vi "CRYGet Foot Switch.vi"(11 "Switch Mode":enum16{"ONESTOP_MODE", "CONTINUE_MODE"}(ring)) -> (3 "bResult":bool)   [LabVIEW 2013]
uses:
  CRYMainGlobal.vi
  Hardware/SubVI/CRY6175APT_Win32.dll
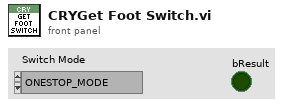
[diagram p1: front panel]
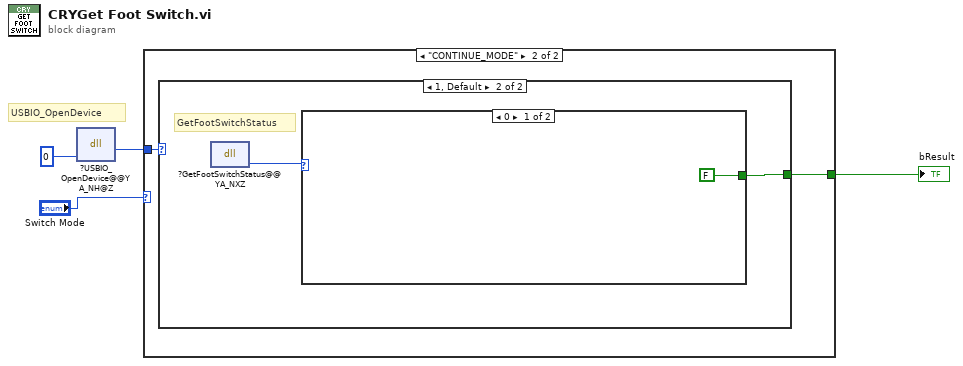
[diagram p0: block diagram]
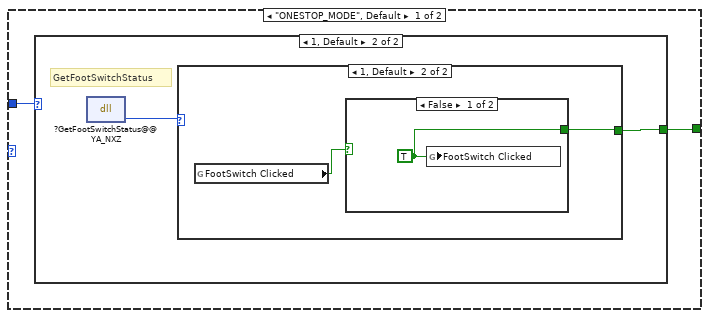
[diagram p2: hidden frame]
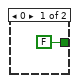
[diagram p3: hidden frame]
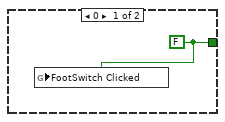
[diagram p4: hidden frame]
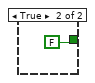
[diagram p5: hidden frame]
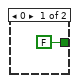
[diagram p6: hidden frame]
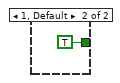
[diagram p7: hidden frame]
diagram:
  # "USBIO_OpenDevice"
  n1 = dll-call lib="D:/A_CRYSoundLab_Work/CRY6181/CRYSystem/Hardware/SubVI/CRY6175APT_Win32.dll" fn="?USBIO_OpenDevice@@YA_NH@Z"("nDevID"=0) -> ("return type"=w3:i32)  [unwired: 4 in, 2 out]
  n2 = case shown="\"CONTINUE_MODE\"" "Switch Mode" {
    tunnel: w3 -> [w5 w16]
    tunnel: [w6 w15] -> w2
    frame "ONESTOP_MODE", Default {
      n3 = case shown="1, Default" w5 {
        tunnel: [FALSE w8] -> w6
        frame 0 {
        }
        frame 1, Default {
          # "GetFootSwitchStatus"
          n4 = dll-call lib="D:/A_CRYSoundLab_Work/CRY6181/CRYSystem/Hardware/SubVI/CRY6175APT_Win32.dll" fn="?GetFootSwitchStatus@@YA_NXZ"() -> ("return type"=w9:i32)  [unwired: 3 in, 2 out]
          n5 = case shown="1, Default" w9 {
            tunnel: [w10 w11] -> w8
            frame 0 {
              w10 = FALSE
              n6 = global write "CRYMainGlobal.vi" "FootSwitch Clicked"(w10) -> ()
            }
            frame 1, Default {
              n7 = global read "CRYMainGlobal.vi" "FootSwitch Clicked"() -> (w12:bool)
              n8 = case shown="False" w12 {
                tunnel: [w13 FALSE] -> w11
                frame False {
                  w13 = TRUE ("FootSwitch Clicked")
                  n9 = global write "CRYMainGlobal.vi" "FootSwitch Clicked"(w13) -> ()
                }
                frame True {
                }
              }
            }
          }
        }
      }
    }
    frame "CONTINUE_MODE" {
      n10 = case shown="1, Default" w16 {
        tunnel: [FALSE w18] -> w15
        frame 0 {
        }
        frame 1, Default {
          # "GetFootSwitchStatus"
          n11 = dll-call lib="D:/A_CRYSoundLab_Work/CRY6181/CRYSystem/Hardware/SubVI/CRY6175APT_Win32.dll" fn="?GetFootSwitchStatus@@YA_NXZ"() -> ("return type"=w19:i32)  [unwired: 3 in, 2 out]
          n12 = case shown="0" w19 {
            tunnel: [FALSE TRUE] -> w18
            frame 0 {
            }
            frame 1, Default {
            }
          }
        }
      }
    }
  }
  "bResult" <- w2
